vi "SingleBitTests.vi"(0 "Connection ID TB":refnum<k5>, 1 "connection ID CC":refnum<k5>, 2 "Ring":i32(ring) items=["DE Bearing Temp Trip", "Drive Ready", "Motor Temp Trip", "NDE Bearing Temp Trip", "Register Mode", "Sync Mode", "MP PRESENT", "EEP PRESENT", "1MHz PRESENT", "DATA VETO 1MHz", "DATA VETO MP", "DATA VETO EEP"], 3 "error in (no error)":errorcluster, 4 "Chopper Serial Number":string="26") -> (5 "String":string, 6 "PASS":bool, 7 "error out":errorcluster)   [LabVIEW 2013]
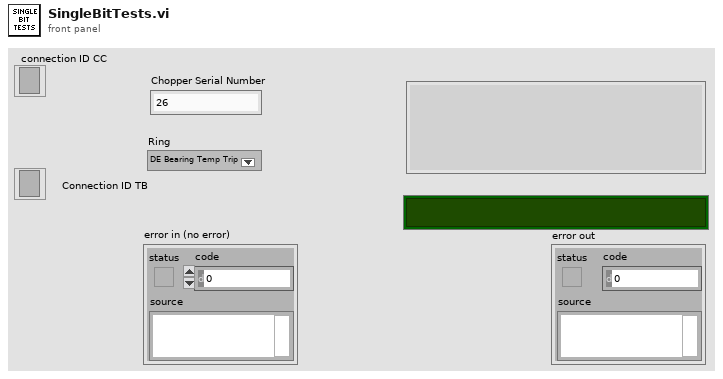
[diagram p1: front panel]
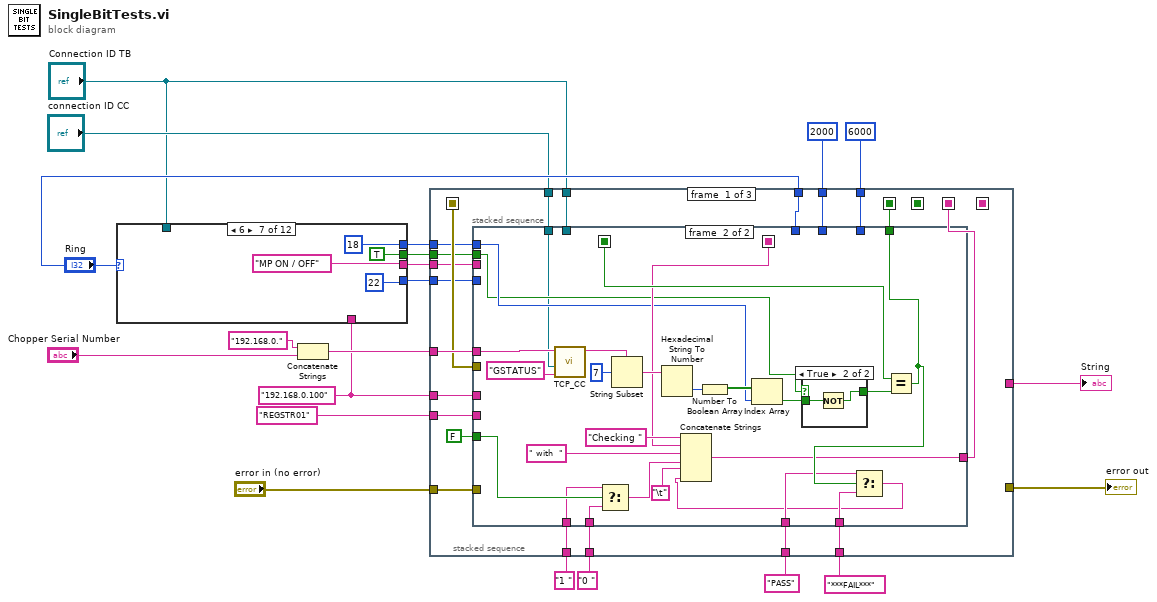
[diagram p0: block diagram]
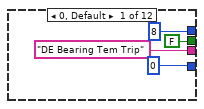
[diagram p2: hidden frame]
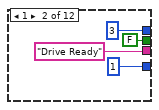
[diagram p3: hidden frame]
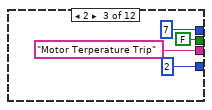
[diagram p4: hidden frame]
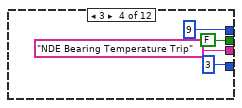
[diagram p5: hidden frame]
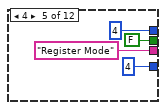
[diagram p6: hidden frame]
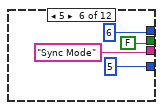
[diagram p7: hidden frame]
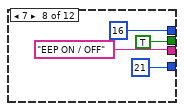
[diagram p8: hidden frame]
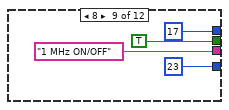
[diagram p9: hidden frame]
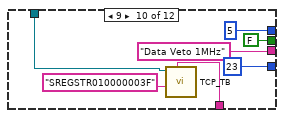
[diagram p10: hidden frame]
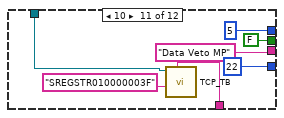
[diagram p11: hidden frame]
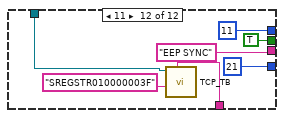
[diagram p12: hidden frame]
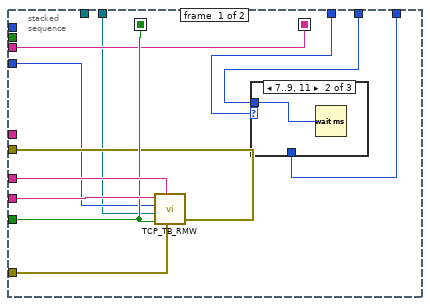
[diagram p13: hidden frame]
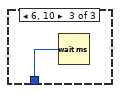
[diagram p15: hidden frame]
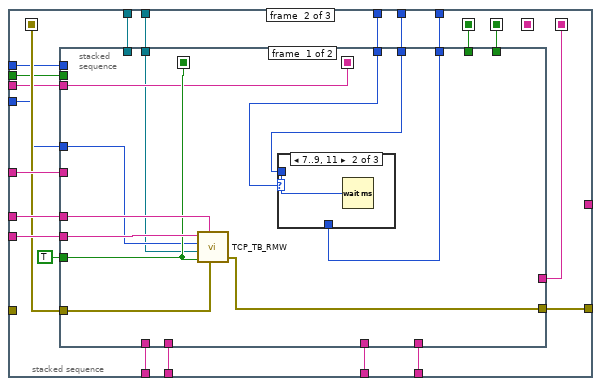
[diagram p17: hidden frame]
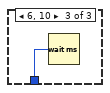
[diagram p19: hidden frame]
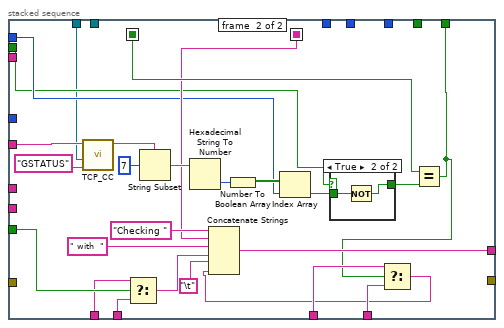
[diagram p20: hidden frame]
diagram:
  w3 = "192.168.0.100" ("TB IP ADDRESS")
  n1 = case shown="6" "Ring" {
    tunnel: [0 ("Bit Bumber") 1 ("Bit Bumber") 2 ("Bit Bumber") 3 ("Bit Bumber") 4 ("Bit Bumber") 5 ("Bit Bumber") 22 ("Bit Bumber") 21 ("Bit Bumber") 23 ("Bit Bumber") 23 ("Bit Bumber") 22 ("Bit Bumber") 21 ("Bit Bumber")] -> w11
    tunnel: [8 ("Bit Bumber") 3 ("Bit Bumber") 7 ("Bit Bumber") 9 ("Bit Bumber") 4 ("Bit Bumber") 6 ("Bit Bumber") 18 ("Bit Bumber") 16 ("Bit Bumber") 17 ("Bit Bumber") 5 ("Bit Bumber") 5 ("Bit Bumber") 11 ("Bit Bumber")] -> w10
    tunnel: [FALSE FALSE FALSE FALSE FALSE FALSE TRUE TRUE TRUE FALSE FALSE TRUE] -> w9
    tunnel: ["DE Bearing Tem Trip" "Drive Ready" "Motor Terperature Trip" "NDE Bearing Temperature Trip" "Register Mode" "Sync Mode" "MP ON / OFF" "EEP ON / OFF" "1 MHz ON/OFF" "Data Veto 1MHz" "Data Veto MP" "EEP SYNC"] -> w8
    tunnel: w3 -> [_ _ _ _ _ _ _ _ _ w60 w67 w74]
    tunnel: "Connection ID TB" -> [_ _ _ _ _ _ _ _ _ w58 w65 w72]
    frame 0, Default {
    }
    frame 1 {
    }
    frame 2 {
    }
    frame 3 {
    }
    frame 4 {
    }
    frame 5 {
    }
    frame 6 {
    }
    frame 7 {
    }
    frame 8 {
    }
    frame 9 {
      n2 = call "TCP_TB.vi"("IP ADDRESS"=w60, "COMMAND"="SREGSTR010000003F", "Connection ID IN"=w58) -> ()  [unwired: 3 in, 3 out]
    }
    frame 10 {
      n3 = call "TCP_TB.vi"("IP ADDRESS"=w67, "COMMAND"="SREGSTR010000003F", "Connection ID IN"=w65) -> ()  [unwired: 3 in, 3 out]
    }
    frame 11 {
      n4 = call "TCP_TB.vi"("IP ADDRESS"=w74, "COMMAND"="SREGSTR010000003F", "Connection ID IN"=w72) -> ()  [unwired: 3 in, 3 out]
    }
  }
  n5 = Concatenate Strings("192.168.0." ("TB IP ADDRESS"), "Chopper Serial Number") -> (w18:string)
  n6 = stacked-sequence {
    seq-local: [w94 _ _] -> [_ w159 w216]
    seq-local: [_ w154 _] -> [_ _ w217]
    seq-local: [w89 _ _] -> [_ _ w214]
    seq-local: [_ w153 _] -> [_ _ w213]
    seq-local: [w88 _ _] -> [_ w152 _]
    tunnel: w3 -> [w99 w163 w209]
    tunnel: "REGSTR01" ("REGISTER") -> [w98 w162 w210]
    tunnel: "error in (no error)" -> [w97 _ _]
    tunnel: w18 -> [w96 w161 _]
    tunnel: "0 " -> [w93 w158 _]
    tunnel: "1 " -> [w92 w157 _]
    tunnel: "PASS" -> [w91 w156 _]
    tunnel: "***FAIL***" -> [w90 w155 _]
    tunnel: [_ _ w212] -> w13
    tunnel: [_ w151 _] -> w12
    tunnel: w11 -> [w87 w147 w207]
    tunnel: w10 -> [w86 w150 _]
    tunnel: w9 -> [w85 w149 _]
    tunnel: w8 -> [w84 w148 _]
    tunnel: "Ring" -> [w81 w146 _]
    tunnel: u32 2000 ("milliseconds to wait") -> [w82 w145 _]
    tunnel: u32 6000 ("milliseconds to wait") -> [w83 w144 _]
    tunnel: "connection ID CC" -> [w80 w143 _]
    tunnel: "Connection ID TB" -> [w79 w142 w206]
    frame #0 {
      n7 = stacked-sequence {
        seq-local: [w107 _] -> [_ w129]
        seq-local: [w104 _] -> [_ w116]
        tunnel: w99 -> [w110 _]
        tunnel: w98 -> [w109 _]
        tunnel: w97 -> [w108 _]
        tunnel: w96 -> [_ w138]
        tunnel: FALSE ("Value 1 (TRUE)") -> [w107 w127]
        tunnel: [_ w121] -> w94
        tunnel: w93 -> [_ w124]
        tunnel: w92 -> [_ w123]
        tunnel: w91 -> [_ w120]
        tunnel: w90 -> [_ w119]
        tunnel: [_ w117] -> w89
        tunnel: [w106 _] -> w88
        tunnel: w87 -> [w105 _]
        tunnel: w86 -> [_ w115]
        tunnel: w85 -> [_ w114]
        tunnel: w84 -> [w104 _]
        tunnel: w83 -> [w103 _]
        tunnel: w82 -> [w102 _]
        tunnel: w81 -> [w101 _]
        tunnel: w80 -> [_ w113]
        tunnel: w79 -> [w100 _]
        frame #0 {
          n8 = call "TCP_TB_RMW.vi"("REGISTER"=w109, "TB IP ADDRESS"=w110, "Bit Bumber"=w105, "Connection ID IN"=w100, "error in (no error)"=w108, "Value 1 (TRUE)"=w107) -> ("error out"=w106:errorcluster)  [unwired: 2 out]
          n9 = case shown="7..9, 11" w101 {
            tunnel: w102 -> [_ w111 _]
            tunnel: w103 -> [_ _ w112]
            frame 0, Default {
            }
            frame 7..9, 11 {
              n10 = Wait (ms)(milliseconds to wait=w111) -> ()  [unwired: 1 out]
            }
            frame 6, 10 {
              n11 = Wait (ms)(milliseconds to wait=w112) -> ()  [unwired: 1 out]
            }
          }
        }
        frame #1 {
          n12 = call "TCP_CC.vi"("COMMAND"="GSTATUS", "connection ID"=w113, "IP ADDRESS"=w138) -> ("The Response:"=w136:string)  [unwired: 1 in, 3 out]
          n13 = Select(t=w123, s=w127, f=w124) -> (s? t:f=w125:string)
          n14 = String Subset(string=w136, offset (0)=7) -> (substring=w135:string)  [unwired: 1 in]
          n15 = Hexadecimal String To Number(string=w135) -> (number=w134:u32)  [unwired: 2 in, 1 out]
          n16 = Number To Boolean Array(number=w134) -> (Boolean array=w133:bool[])
          n17 = Index Array(array=w133, index=w115) -> (element=w131:bool)
          n18 = case shown="True" w114 {
            tunnel: [w139 w140] -> w130
            tunnel: w131 -> [w139 w141]
            frame False {
            }
            frame True {
              n19 = Not(x=w141) -> (.not. x?=w140:bool)
            }
          }
          n20 = Equal?(x=w129, y=w130) -> (x = y?=w121:bool)
          n21 = Select(t=w120, s=w121, f=w119) -> (s? t:f=w118:string)
          n22 = Concatenate Strings("Checking ", w116, " with  ", w125, "\t", w118) -> (w117:string)
        }
      }
    }
    frame #1 {
      n23 = stacked-sequence {
        seq-local: [w171 _] -> [_ w193]
        seq-local: [w169 _] -> [_ w191]
        tunnel: w163 -> [w174 _]
        tunnel: w162 -> [w173 _]
        tunnel: w152 -> [w172 _]
        tunnel: w161 -> [_ w202]
        tunnel: TRUE ("Value 1 (TRUE)") -> [w171 w190]
        tunnel: w159 -> [_ _]
        tunnel: w158 -> [_ w187]
        tunnel: w157 -> [_ w186]
        tunnel: w156 -> [_ w184]
        tunnel: w155 -> [_ w183]
        tunnel: [_ w181] -> w153
        tunnel: [_ w180] -> w154
        tunnel: [w170 _] -> w151
        tunnel: w150 -> [_ w179]
        tunnel: w149 -> [_ w178]
        tunnel: w148 -> [w169 _]
        tunnel: w147 -> [w168 _]
        tunnel: w146 -> [w167 _]
        tunnel: w145 -> [w166 _]
        tunnel: w144 -> [w165 _]
        tunnel: w143 -> [_ w177]
        tunnel: w142 -> [w164 _]
        frame #0 {
          n24 = call "TCP_TB_RMW.vi"("REGISTER"=w173, "TB IP ADDRESS"=w174, "Bit Bumber"=w168, "Connection ID IN"=w164, "error in (no error)"=w172, "Value 1 (TRUE)"=w171) -> ("error out"=w170:errorcluster)  [unwired: 2 out]
          n25 = case shown="7..9, 11" w167 {
            tunnel: w166 -> [_ w175 _]
            tunnel: w165 -> [_ _ w176]
            frame 0, Default {
            }
            frame 7..9, 11 {
              n26 = Wait (ms)(milliseconds to wait=w175) -> ()  [unwired: 1 out]
            }
            frame 6, 10 {
              n27 = Wait (ms)(milliseconds to wait=w176) -> ()  [unwired: 1 out]
            }
          }
        }
        frame #1 {
          n28 = call "TCP_CC.vi"("COMMAND"="GSTATUS", "connection ID"=w177, "IP ADDRESS"=w202) -> ("The Response:"=w200:string)  [unwired: 1 in, 3 out]
          n29 = Select(t=w186, s=w190, f=w187) -> (s? t:f=w188:string)
          n30 = String Subset(string=w200, offset (0)=7) -> (substring=w199:string)  [unwired: 1 in]
          n31 = Hexadecimal String To Number(string=w199) -> (number=w198:u32)  [unwired: 2 in, 1 out]
          n32 = Number To Boolean Array(number=w198) -> (Boolean array=w197:bool[])
          n33 = Index Array(array=w197, index=w179) -> (element=w195:bool)
          n34 = case shown="True" w178 {
            tunnel: [w203 w204] -> w194
            tunnel: w195 -> [w203 w205]
            frame False {
            }
            frame True {
              n35 = Not(x=w205) -> (.not. x?=w204:bool)
            }
          }
          n36 = Equal?(x=w193, y=w194) -> (x = y?=w180:bool)
          n37 = Select(t=w184, s=w180, f=w183) -> (s? t:f=w182:string)
          n38 = Concatenate Strings("Checking ", w191, " with  ", w188, "\t", w182) -> (w181:string)
        }
      }
    }
    frame #2 {
      w211 = "\r"
      n39 = call "TCP_TB_RMW.vi"("REGISTER"=w210, "TB IP ADDRESS"=w209, "Bit Bumber"=w207, "Connection ID IN"=w206, "Value 1 (TRUE)"=FALSE) -> ()  [unwired: 1 in, 3 out]
      n40 = Concatenate Strings(w214, w211, w213, w211) -> (w212:string)
      n41 = And(x=w217, y=w216) -> (x .and. y?=→"PASS":bool)
    }
  }
  "String" <- w13
  "error out" <- w12
